vi "Error Module.vi"(7 "Command (Handle Errors":T4=enum."Handle Errors", 8 "error in":errorcluster, 9 "dynamic event queue reference":T3, 10 "User Interface Queue Reference":T2, 11 "User Event Queue Refence":T1) -> (0 "error out":errorcluster, 2 "status":bool)   [LabVIEW 2011]
doc: "Controls access to the Cue data."
uses:
  Error Module Action.ctl
  Controls/Dynamic Event Queue Reference.ctl
  Controls/User Interface Queue Reference.ctl
  Controls/User Interface Control.ctl
  Controls/User Interface Action.ctl
  Controls/User Event Queue Reference.ctl
  Controls/User Event Control.ctl
  Controls/User Event Action.ctl
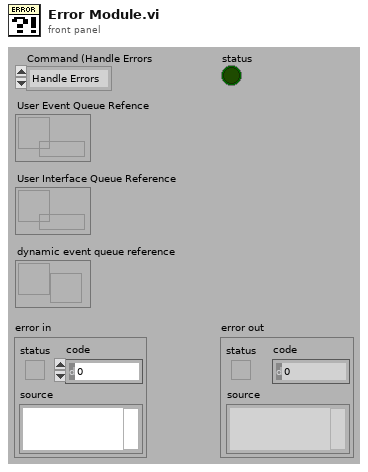
[diagram p1: front panel]
types:
  T1 = typedef "User Event Queue Reference.ctl" = refnum<queue>
  T2 = typedef "User Interface Queue Reference.ctl" = refnum<queue>
  T3 = typedef "Dynamic Event Queue Reference.ctl" = refnum<user-event>
  T4 = typedef "Error Module Action.ctl" = enum16{"Initialize", "Handle Errors", "Report Errors"}
  T5 = typedef "User Interface Control.ctl" = cluster{"action":T6, "data1":variant, "data2":variant}
  T6 = typedef "User Interface Action.ctl" = enum16{"Initialize", "Data Acquisition Disable", "Data View Disable", "Sample Set", "Sample Set 2D Data", "Sample Set x0 & dx", "Sample Add", "Sample Set Cursor", "Sample Set Offset & Multiplier", "Sample Set Axis Labels", "Sample Parameters Disabled", "Sample Parameters Update", "Run Update", "Run Set Offset & Multiplier", "Run Set Axis Labels", "Run Set Cursor", "Run Set Disabled", "Run Parameters Update", "Run Parameters Disabled", "Run Number Set", "Run Number Set Range", "Run Number Set Disabled", "Sample Number Set", "Sample Number Set Range", "Notes Set Value", "Update Plot", "Set Plot Parameters", "Update Concentration Plot", "Time Set", "Clear DAQ Display", "Clear Analysis Display", "Status Bar Set", "Progress Bar Set", "Display Mode Set", "Experiment Type Set", "Analysis Plot Average Set", "Stop"}
  T7 = typedef "User Event Control.ctl" = cluster{"action":T8, "data":variant}
  T8 = typedef "User Event Action.ctl" = enum16{"Program Initialization", "Device Connections", "Device Settings", "Options", "DAQ Init", "PID Sample Test", "PID with PS Challenge", "PID with MFC Challenge", "Multimeter Sample Test", "Multimeter with MFC Challenge", "DAQ Stop", "Open Data File", "View Data File", "Change Display Mode", "Load INL PID Run Data", "Load Baseline-Mocon PID Data", "Load Multimeter Data", "Set Channel Sample", "Key Down", "Add Spectrum to Plot", "Add History to Plot", "Export History to Excel", "Clear Plots", "Save Plot", "Save Spectral Variable", "History Cursor Release", "Analysis Plot Cursor Release", "Program Deinitialization"}
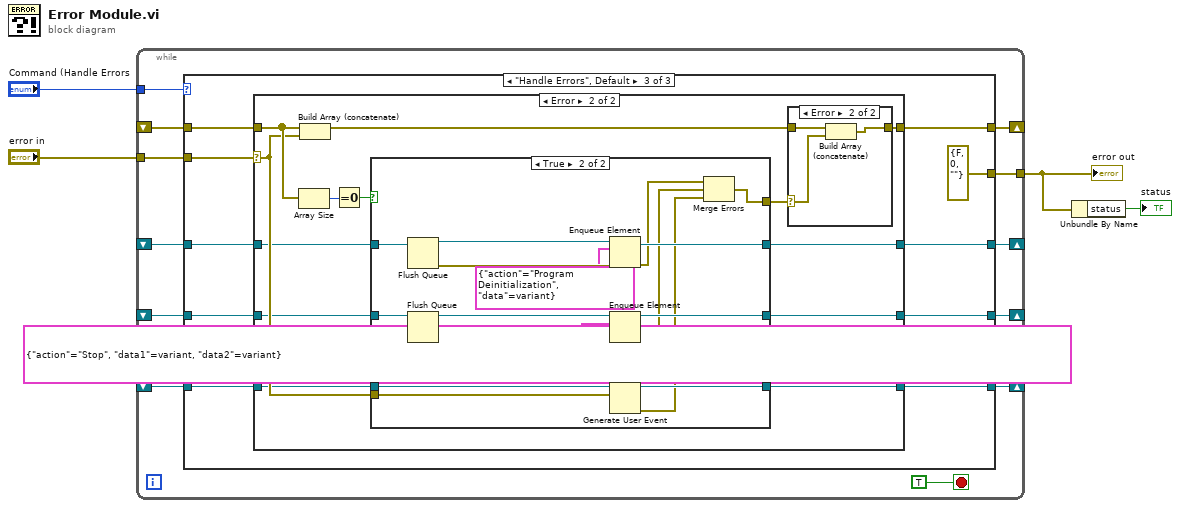
[diagram p0: block diagram]
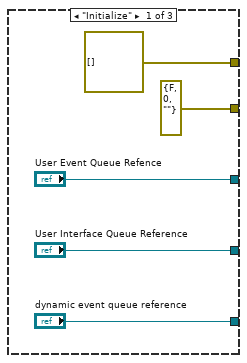
[diagram p2: hidden frame]
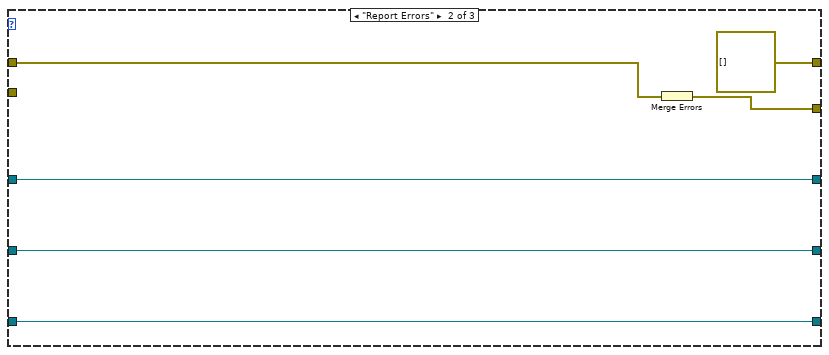
[diagram p3: hidden frame]
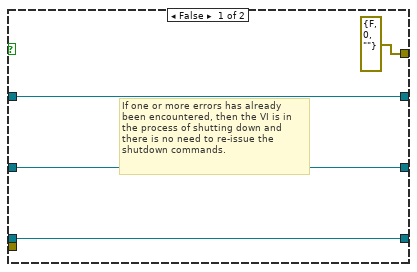
[diagram p6: hidden frame]
diagram:
  n1 = while {
    shift-right: [w12] -> _
    shift-left: _ -> [w14]
    tunnel: "error in" -> [w15]
    tunnel: "Command (Handle Errors" -> [w13]
    tunnel: [w11] -> w2
    shift-right: [w5] -> _
    shift-left: _ -> [w10]
    shift-right: [w6] -> _
    shift-left: _ -> [w9]
    shift-right: [w7] -> _
    shift-left: _ -> [w8]
    stop <- TRUE stop-if-true
    n2 = case shown="\"Handle Errors\", Default" w13 {
      tunnel: w15 -> [_ _ w37]
      tunnel: [errorcluster[] [] errorcluster[] [] w35] -> w12
      tunnel: w14 -> [_ w26 w36]
      tunnel: [errorcluster {"status"=FALSE, "code"=0, "source"=""} ("error out") w27 errorcluster {"status"=FALSE, "code"=0, "source"=""} ("error out")] -> w11
      tunnel: w10 -> [_ w25 w33]
      tunnel: w9 -> [_ w24 w32]
      tunnel: w8 -> [_ w23 w31]
      tunnel: ["dynamic event queue reference" w23 w28] -> w7
      tunnel: ["User Interface Queue Reference" w24 w29] -> w6
      tunnel: ["User Event Queue Refence" w25 w30] -> w5
      frame "Initialize" {
      }
      frame "Report Errors" {
        n3 = Merge Errors(w26) -> (w27:errorcluster)
      }
      frame "Handle Errors", Default {
        n4 = case shown="Error" w37 {
          selector: w37 -> [_ w48]
          tunnel: [w41 w50] -> w35
          tunnel: w36 -> [w41 w54]
          tunnel: w33 -> [w40 w47]
          tunnel: w32 -> [w39 w46]
          tunnel: w31 -> [w38 w45]
          tunnel: [w38 w44] -> w28
          tunnel: [w39 w43] -> w29
          tunnel: [w40 w42] -> w30
          frame No Error {
          }
          frame Error {
            n5 = Array Size(array=w54) -> (size(s)=w52:i32)
            n6 = Build Array (concatenate)(w54, w48) -> (w51:errorcluster[])
            n7 = Equal To 0?(x=w52) -> (x = 0?=w53:bool)
            n8 = case shown="True" w53 {
              tunnel: [errorcluster {"status"=FALSE, "code"=0, "source"=""} ("error out") w68] -> w49
              tunnel: w48 -> [_ w72]
              tunnel: w47 -> [w61 w79]
              tunnel: w46 -> [w60 w78]
              tunnel: w45 -> [w59 w73]
              tunnel: [w59 w71] -> w44
              tunnel: [w60 w70] -> w43
              tunnel: [w61 w69] -> w42
              frame False {
                # "If one or more errors has already \nbeen encountered, then the VI is in \nthe process of shutting down and \nthere is no need to re-issue the \nshutdown commands."
              }
              frame True {
                n9 = Flush Queue(queue=w79) -> (queue out=w77:T1, error out=w74:errorcluster)  [unwired: 1 in, 1 out]
                n10 = Flush Queue(queue=w78) -> (queue out=w76:T2, error out=w75:errorcluster)  [unwired: 1 in, 1 out]
                n11 = Enqueue Element(queue=w77, element=T7 {"action"=enum."Program Deinitialization", "data"=variant} ("User Event Control"), error in (no error)=w74) -> (queue out=w69:T1, error out=w67:errorcluster)  [unwired: 1 in, 1 out]
                n12 = Enqueue Element(queue=w76, element=T5 {"action"=enum."Stop", "data1"=variant, "data2"=variant} ("User Interface Control"), error in (no error)=w75) -> (queue out=w70:T2, error out=w66:errorcluster)  [unwired: 1 in, 1 out]
                n13 = Generate User Event(user event=w73, event data cluster=w72) -> (user event out=w71:T3, error out=w65:errorcluster)  [unwired: 1 in]
                n14 = Merge Errors(w67, w66, w65) -> (w68:errorcluster)
              }
            }
            n15 = case shown="Error" w49 {
              selector: w49 -> [_ w56]
              tunnel: w51 -> [w55 w58]
              tunnel: [w55 w57] -> w50
              frame No Error {
              }
              frame Error {
                n16 = Build Array (concatenate)(w58, w56) -> (w57:errorcluster[])
              }
            }
          }
        }
      }
    }
  }
  "error out" <- w2
  n17 = Unbundle By Name(w2) -> ("status"=→"status":bool)
